vi "_TangoErrors.vi"() -> (0 "Tango Error codes":i32[](array[numeric])=[-1], 1 "Tango error descs":string[](array[string])=["Tango Error"])   [LabVIEW 2014, in "tango.lvlib"]
uses:
  tango.lvlib
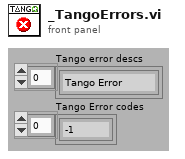
[diagram p1: front panel]
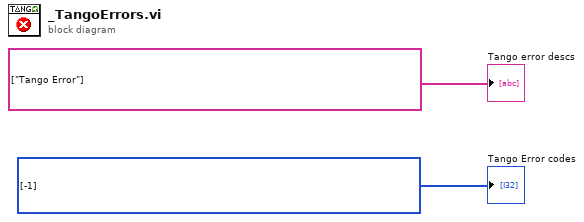
[diagram p0: block diagram]
diagram:
  "Tango error descs" <- string[] ["Tango Error"]
  "Tango Error codes" <- i32[] [-1] ("[user-defined codes]")
